vi "Solenoid With Compressor.vi"() -> ()   [LabVIEW 2025]
doc: "Solenoid With Compressor Example \n\nThis example shows how to control a compressor with a solenoid.\n\nThis example works with the PCM (Pneumatic Control Module) communicating with the roboRIO over CAN bus. The PCM must also be supplied with 12V DC from the PDP (Power Distribution Panel).\n\nThe Compressor, Pressure Switch, and Solenoid are all wired to the PCM \n\nThis example expects a USB cable connected from your development PC to the Type B USB Jack (next to the power input) on the roboRIO.\n\nThis example expects the Driver Station to be running."
uses:
  <vilib>/Rock Robotics/WPI/Solenoid/WPI_SolenoidChannel.ctl
  <vilib>/Rock Robotics/WPI/Solenoid/WPI_SolenoidValue.ctl
  <vilib>/Rock Robotics/WPI/Solenoid/WPI_SolenoidOpenSingle.vi
  <vilib>/Rock Robotics/WPI/Solenoid/WPI_SolenoidGetEnum.vi
  <vilib>/Rock Robotics/WPI/Solenoid/WPI_SolenoidSetEnum.vi
panel:
  out "Value":T1
  in  "Select a PD device by clicking on the image below":u16(ring) items=["CTRE Pneumatic Module", "REV Pneumatics Hub"]
  in  "Solenoid Channel":T2
  out "Compressor Monitoring?":bool
  in  "stop":bool
  in  "Solenoid":bool
  # "Wiring Diagram"
  # "Set this input before running."
  # "This can be set while running."
  # "Output information"
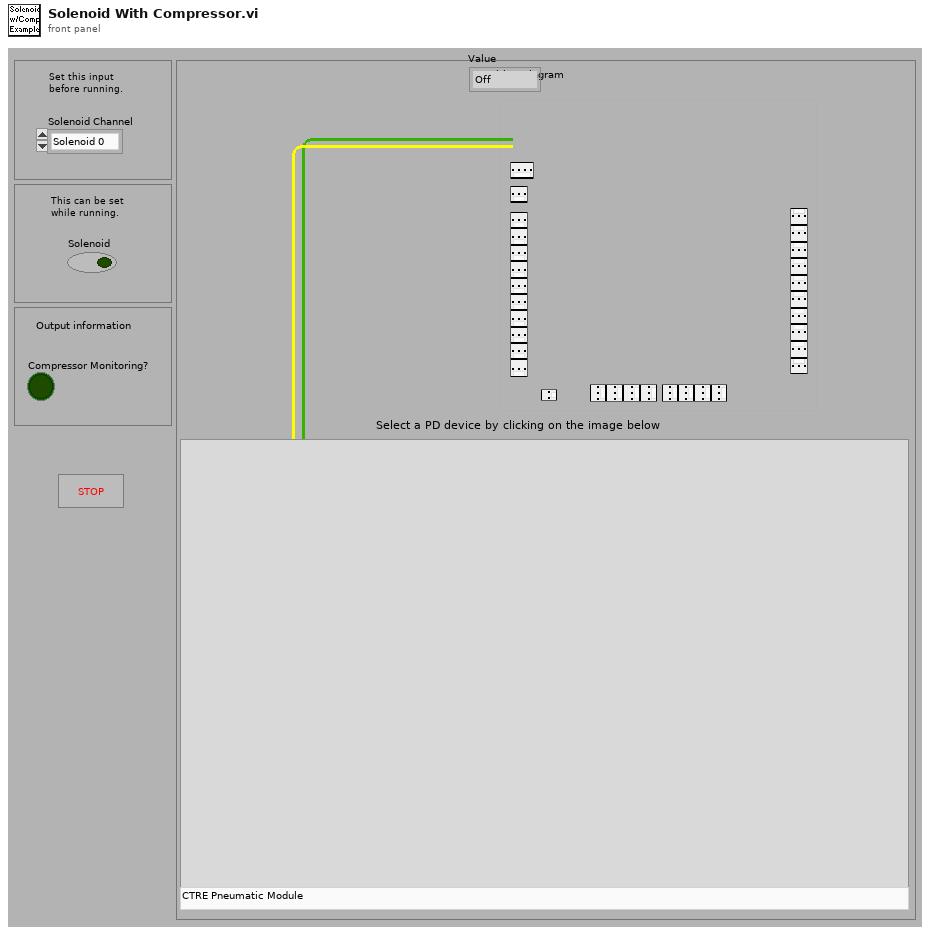
[diagram p1: front panel]
types:
  T1 = typedef "WPI_SolenoidValue.ctl" = enum16{"Off", "On", "Forward", "Reverse"}
  T2 = typedef "WPI_SolenoidChannel.ctl" = enum8{"Solenoid 0", "Solenoid 1", "Solenoid 2", "Solenoid 3", "Solenoid 4", "Solenoid 5", "Solenoid 6", "Solenoid 7", "Solenoid 8", "Solenoid 9", "Solenoid 10", "Solenoid 11", "Solenoid 12", "Solenoid 13", "Solenoid 14", "Solenoid 15", "Invalid"}
  T3 = typedef "WPI_CompressorDevRef.ctl" = cluster{"DevStatus":errorcluster, "Pneumatics Control Module":u8}
  T4 = typedef "WPI_SolenoidDevRef.ctl" = cluster{"DevStatus":errorcluster, "Pneumatics Control Module":u8, "Forward Solenoid Channel":T2, "Reverse Solenoid Channel":T2}
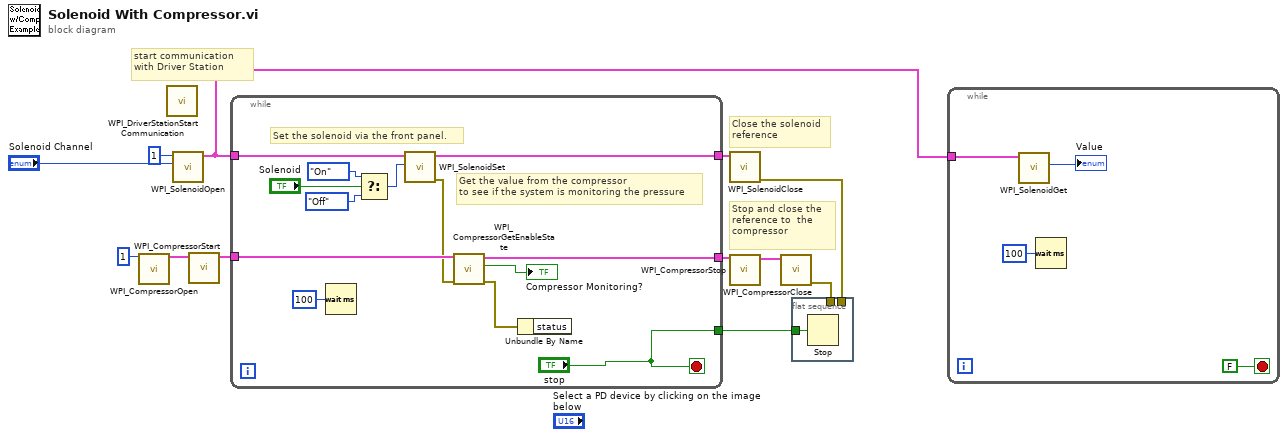
[diagram p0: block diagram]
diagram:
  # "start communication with Driver Station"
  # "Close the solenoid\nreference"
  # "Stop and close the reference to  the compressor"
  n1 = call <vilib>:"WPI_CompressorOpen.vi"("Pneumatics device (def)"=u8 1 ("Pneumatics device (0)")) -> ("CompressorDevRef"=w7:T3)  [unwired: 13 in, 1 out]
  n2 = call <vilib>:"WPI_DriverStationStart Communication.vi"() -> ()  [unwired: 3 in, 9 out]
  n3 = call-poly <vilib>:"WPI_SolenoidOpen.vi"("Solenoid Channel"="Solenoid Channel", "Pneumatics Device (def)"=u8 1 ("Pneumatics Control Module (0)")) -> ("SolenoidDevRef"=w1:T4)  [unwired: 1 in, 8 out]
  n4 = call <vilib>:"WPI_CompressorStart.vi"("CompressorDevRef"=w7) -> ("CompressorDevRef"=w9:T3)  [unwired: 2 in, 8 out]
  n5 = while {
    tunnel: w1 -> [w25]
    tunnel: [w14] -> w11
    tunnel: w9 -> [w24]
    tunnel: [w23] -> w8
    tunnel: ["stop"] -> w4
    stop <- "stop" stop-if-true
    # "Get the value from the compressor \nto see if the system is monitoring the pressure"
    # "Set the solenoid via the front panel."
    n6 = Wait (ms)(milliseconds to wait=u32 100) -> ()  [unwired: 1 out]
    n7 = Select(t=WPI_SolenoidValue."On" ("Value"), s="Solenoid", f=WPI_SolenoidValue."Off" ("Value")) -> (s? t:f=w15:T1)
    n8 = call-poly <vilib>:"WPI_SolenoidSet.vi"("Value"=w15, "SolenoidDevRef"=w25) -> ("error out"=w21:errorcluster, "SolenoidDevRef"=w14:T4)  [unwired: 1 in, 7 out]
    n9 = call <vilib>:"WPI_CompressorGetEnableState.vi"("error in (no error)"=w21, "CompressorDevRef"=w24) -> ("error out"=w19:errorcluster, "Enabled"=→"Compressor Monitoring?":bool, "CompressorDevRef"=w23:T3)  [unwired: 7 out]
    n10 = Unbundle By Name(w19) -> ()  [unwired: 1 out]
  }
  n11 = call <vilib>:"WPI_SolenoidClose.vi"("SolenoidDevRef"=w11) -> ("error out"=w5:errorcluster)  [unwired: 1 in, 9 out]
  n12 = call <vilib>:"WPI_CompressorStop.vi"("CompressorDevRef"=w8) -> ("CompressorDevRef"=w10:T3)  [unwired: 1 in, 9 out]
  n13 = call <vilib>:"WPI_CompressorClose.vi"("CompressorDevRef"=w10) -> ("error out"=w6:errorcluster)  [unwired: 1 in, 9 out]
  n14 = flat-sequence {
    tunnel: w6 -> [_]
    tunnel: w5 -> [_]
    tunnel: w4 -> [w26]
    frame #0 {
      n15 = Stop(stop? (T)=w26) -> ()
    }
  }
  n16 = while {
    tunnel: w1 -> [w29]
    stop <- FALSE stop-if-true
    n17 = call-poly <vilib>:"WPI_SolenoidGet.vi"("SolenoidDevRef"=w29) -> ("Value"=→"Value":T1)  [unwired: 8 in, 2 out]
    n18 = Wait (ms)(milliseconds to wait=u32 100) -> ()  [unwired: 1 out]
  }
